vi "RB2 parse  time string.vi"(0 "Nav String":string="$,A,43,13,230,B,10,20,120,C,10,10,330,D,14,36,110,T,08,12,234,S,12,6,123\r") -> (1 "output cluster":cluster{i32, i32, i32}, 2 "Valid?":bool)   [LabVIEW 2012]
doc: "This VI will parse the Tug navigation string for the time; it returns three values: hrs, mins, seconds."
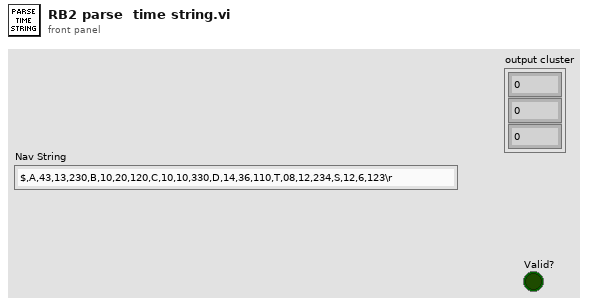
[diagram p1: front panel]
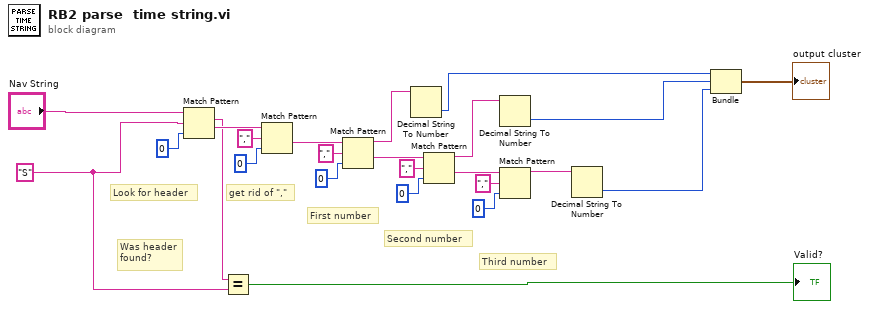
[diagram p0: block diagram]
diagram:
  w4 = "S" ("Header")
  # "Was header\nfound?"
  # "Third number"
  # "Second number"
  # "First number"
  # "get rid of \",\""
  # "Look for header"
  n1 = Match Pattern(string="Nav String", regular expression=w4, offset (0)=0) -> (match substring=w5:string, after substring=w9:string)  [unwired: 2 out]
  n2 = Equal?(x=w5, y=w4) -> (x = y?=→"Valid?":bool)
  n3 = Match Pattern(string=w9, regular expression=",", offset (0)=0) -> (after substring=w10:string)  [unwired: 3 out]
  n4 = Match Pattern(string=w10, regular expression=",", offset (0)=0) -> (before substring=w21:string, after substring=w17:string)  [unwired: 2 out]
  n5 = Decimal String To Number(string=w21) -> (number=w8:i32)  [unwired: 2 in, 1 out]
  n6 = Match Pattern(string=w17, regular expression=",", offset (0)=0) -> (before substring=w18:string, after substring=w13:string)  [unwired: 2 out]
  n7 = Decimal String To Number(string=w18) -> (number=w2:i32)  [unwired: 2 in, 1 out]
  n8 = Match Pattern(string=w13, regular expression=",", offset (0)=0) -> (before substring=w14:string)  [unwired: 3 out]
  n9 = Decimal String To Number(string=w14) -> (number=w7:i32)  [unwired: 2 in, 1 out]
  n10 = Bundle(w8, w2, w7) -> (→"output cluster":cluster{i32, i32, i32})  [unwired: 1 in]
